vi "Queue Driver.vi"(0 "Name":string, 5 "State":string, 7 "States[]":string[](array[string]), 11 "error in (no error)":errorcluster, 13 "Queue Operations":T1) -> (4 "Dequeued State":string, 15 "error out":errorcluster)   [LabVIEW 2021]
uses:
  controls/Queue Operations.ctl
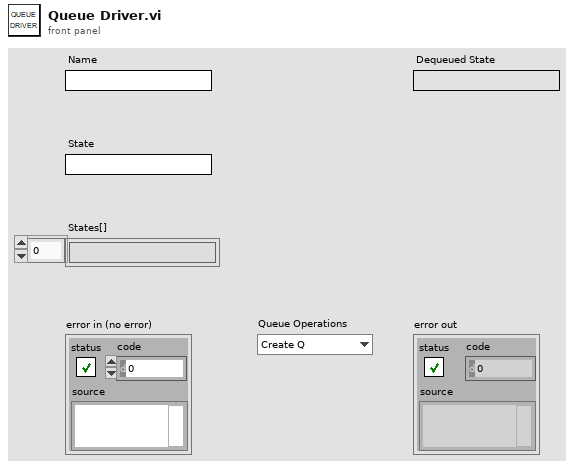
[diagram p1: front panel]
types:
  T1 = typedef "Queue Operations.ctl" = enum16{"Create Q", "Enqueue", "Enqueue N", "Dequeue", "Flush", "Release"}
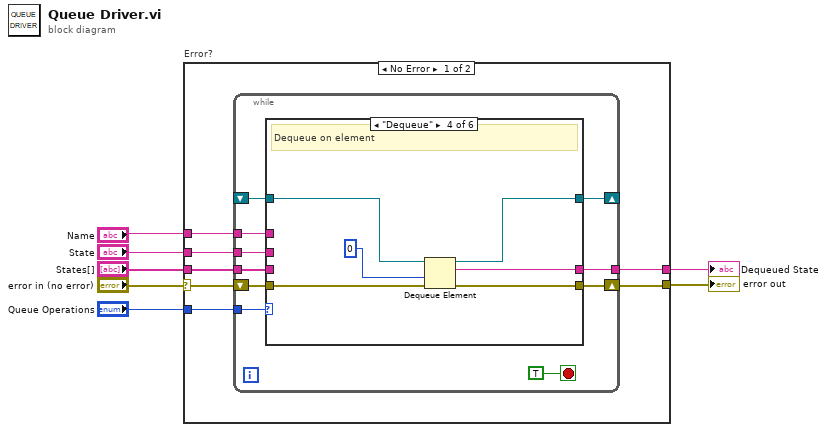
[diagram p0: block diagram]
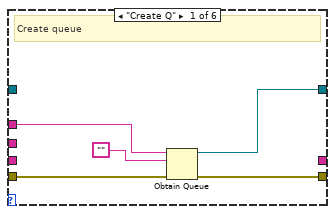
[diagram p2: hidden frame]
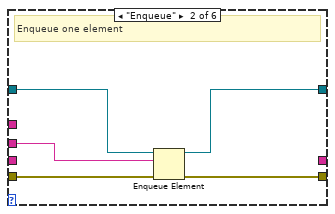
[diagram p3: hidden frame]
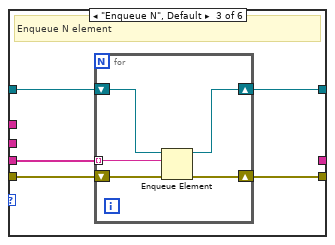
[diagram p4: hidden frame]
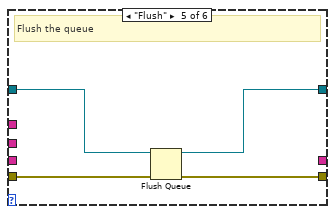
[diagram p5: hidden frame]
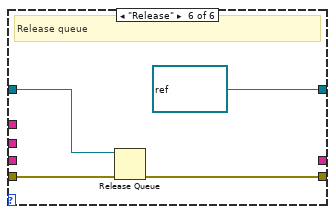
[diagram p6: hidden frame]
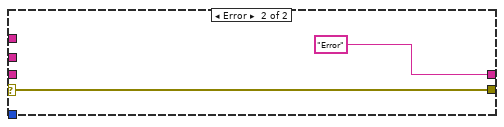
[diagram p7: hidden frame]
diagram:
  n1 = case "Error?" shown="No Error" "error in (no error)" {
    selector: "error in (no error)" -> [w14 w60]
    tunnel: [w12 w60] -> w6
    tunnel: "Queue Operations" -> [w13 _]
    tunnel: "Name" -> [w11 _]
    tunnel: "State" -> [w10 _]
    tunnel: "States[]" -> [w9 _]
    tunnel: [w8 "Error"] -> w1
    frame No Error {
      n2 = while {
        shift-right: [w21] -> w12
        shift-left: w14 -> [w23]
        tunnel: w13 -> [w22]
        shift-right: [w20] -> _
        shift-left: _ -> [w18]
        tunnel: w11 -> [w19]
        tunnel: w10 -> [w17]
        tunnel: w9 -> [w16]
        tunnel: [w15] -> w8
        stop <- TRUE stop-if-true
        n3 = case shown="\"Dequeue\"" w22 {
          tunnel: w23 -> [w29 w34 w39 w50 w54 w58]
          tunnel: [w28 w32 w35 w49 w52 w56] -> w21
          tunnel: [w27 w31 w36 w47 w51 refnum<queue> refnum ("queue out")] -> w20
          tunnel: w19 -> [w26 _ _ _ _ _]
          tunnel: w18 -> [_ w33 w38 w48 w53 w57]
          tunnel: w17 -> [_ w30 _ _ _ _]
          tunnel: w16 -> [_ _ w37 _ _ _]
          tunnel: [_ _ _ w46 _ _] -> w15
          frame "Create Q" {
            # "Create queue"
            n4 = Obtain Queue(name (unnamed)=w26, element data type="", error in (no error)=w29) -> (queue out=w27:refnum<queue>, error out=w28:errorcluster)  [unwired: 2 in, 1 out]
          }
          frame "Enqueue" {
            # "Enqueue one element"
            n5 = Enqueue Element(queue=w33, element=w30, error in (no error)=w34) -> (queue out=w31:refnum<queue>, error out=w32:errorcluster)  [unwired: 1 in, 1 out]
          }
          frame "Enqueue N", Default {
            # "Enqueue N element"
            n6 = for {
              shift-right: [w43] -> w35
              shift-left: w39 -> [w44]
              shift-right: [w40] -> w36
              shift-left: w38 -> [w42]
              tunnel: w37 -> [w41] mode=indexing
              n7 = Enqueue Element(queue=w42, element=w41, error in (no error)=w44) -> (queue out=w40:refnum<queue>, error out=w43:errorcluster)  [unwired: 1 in, 1 out]
            }
          }
          frame "Dequeue" {
            # "Dequeue on element"
            n8 = Dequeue Element(queue=w48, timeout in ms (-1)=0, error in (no error)=w50) -> (queue out=w47:refnum<queue>, element=w46:string, error out=w49:errorcluster)  [unwired: 1 out]
          }
          frame "Flush" {
            # "Flush the queue"
            n9 = Flush Queue(queue=w53, error in (no error)=w54) -> (queue out=w51:refnum<queue>, error out=w52:errorcluster)  [unwired: 1 out]
          }
          frame "Release" {
            # "Release queue"
            n10 = Release Queue(queue=w57, error in (no error)=w58) -> (error out=w56:errorcluster)  [unwired: 1 in, 2 out]
          }
        }
      }
    }
    frame Error {
    }
  }
  "error out" <- w6
  "Dequeued State" <- w1
